vi "Frequency Calculator.vi"(10 "Digitizing Parameters":T1={"Numbers of Samples"=100, "Sampling Frequency"=1000.0}) -> (2 "Frequency":dbl[](array[numeric]))   [LabVIEW 2017]
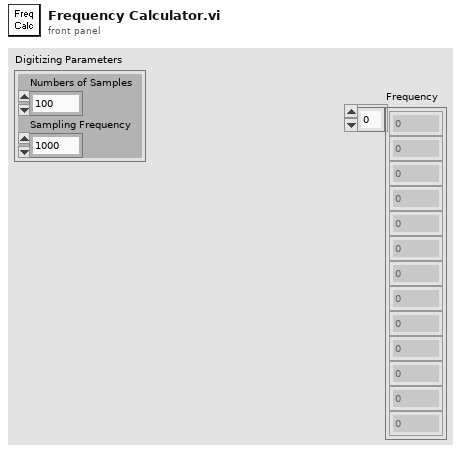
[diagram p1: front panel]
types:
  T1 = cluster{"Numbers of Samples":i32, "Sampling Frequency":dbl}
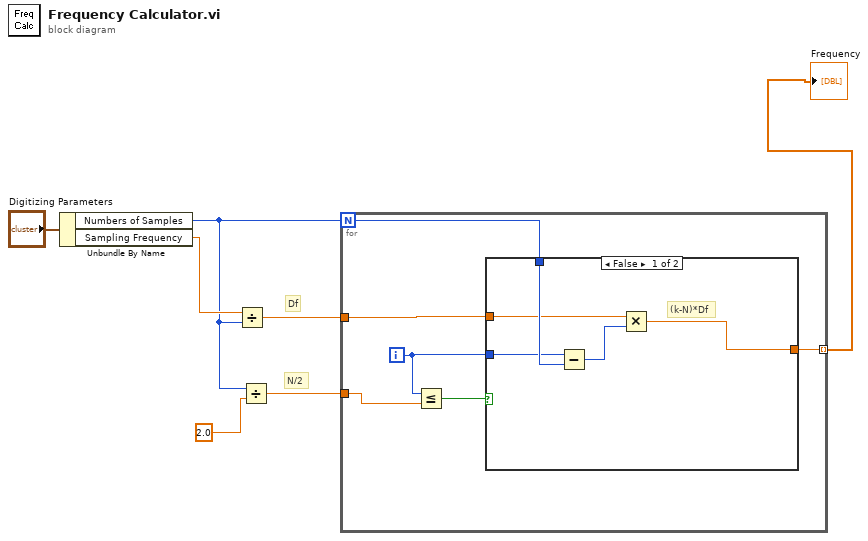
[diagram p0: block diagram]
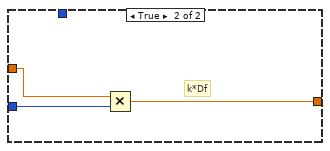
[diagram p2: hidden frame]
diagram:
  # "N/2"
  # "Df"
  n1 = Unbundle By Name("Digitizing Parameters") -> ("Numbers of Samples"=w4:i32, "Sampling Frequency"=w6:dbl)
  n2 = Divide(x=w6, y=w4) -> (x/y=w5:dbl)
  n3 = Divide(x=w4, y=2.0) -> (x/y=w3:dbl)
  n4 = for {
    N: w4 -> [w10]
    tunnel: w5 -> [w12]
    tunnel: w3 -> [w8]
    tunnel: [w11] -> w2 mode=indexing
    i -> [w9]
    n5 = Less Or Equal?(x=w9, y=w8) -> (x <= y?=w13:bool)
    n6 = case shown="False" w13 {
      tunnel: w12 -> [w16 w20]
      tunnel: w9 -> [w17 w21]
      tunnel: [w14 w19] -> w11
      tunnel: w10 -> [w18 _]
      frame False {
        # "(k-N)*Df"
        n7 = Subtract(x=w17, y=w18) -> (x-y=w15:i32)
        n8 = Multiply(x=w16, y=w15) -> (x*y=w14:dbl)
      }
      frame True {
        # "k*Df"
        n9 = Multiply(x=w20, y=w21) -> (x*y=w19:dbl)
      }
    }
  }
  "Frequency" <- w2
